vi "LAC Cmd103_Batch Setting_ver2.vi"(6 "R/W (F:Read)":bool, 7 "timeout(ms)":u32=500, 8 "error in":errorcluster, 9 "setting_items":T1={"binary_lvl"=1600, "noise_lvl"=1600, "LM_HiLimit"=1600, "LM_LoLimit"=1600, "LM_Judge"=0, "LM_Judge type"=0, "Circle-radius"=0.0, "Rect-XL"=0.0, "Rect-XH"=0.0, "Rect-YH"=0.0, "Rect-YL"=0.0, "Circle-radius 2"=0.0, "Off-X"=0.0, "Off-Y"=0.0, "Label mode"=64, "Numbering"=64, "Judge label"=64, "Max spot"=3, "Center cal_method"=64, "Average"=64, "Eff Spot mode"=64, "Spot pixel HiLim"=64, "Spot pixel LoLim"=64}, 11 "VISA name in":refnum<visa-resource-name>) -> (0 "error out":errorcluster, 1 "read buffer":string, 3 "VISA name out":refnum<visa-resource-name>)   [LabVIEW 2018]
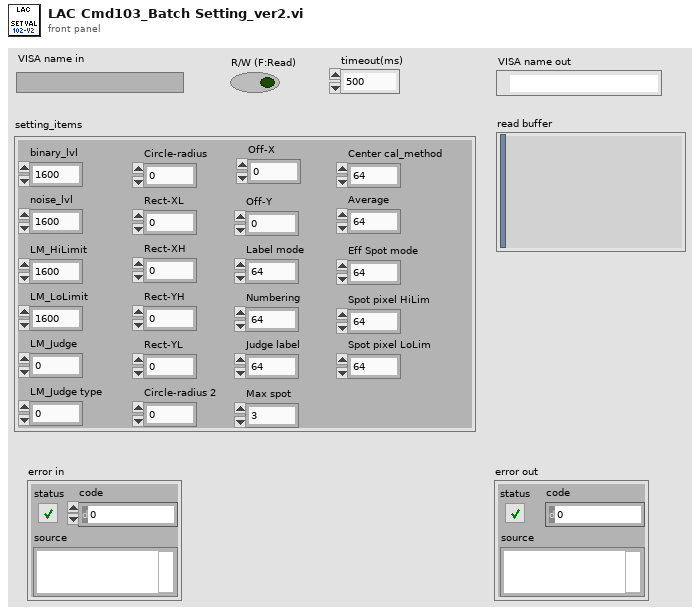
[diagram p1: front panel]
types:
  T1 = cluster{"binary_lvl":u16, "noise_lvl":u16, "LM_HiLimit":u16, "LM_LoLimit":u16, "LM_Judge":u8, "LM_Judge type":u8, "Circle-radius":dbl, "Rect-XL":dbl, "Rect-XH":dbl, "Rect-YH":dbl, "Rect-YL":dbl, "Circle-radius 2":dbl, "Off-X":dbl, "Off-Y":dbl, "Label mode":u8, "Numbering":u8, "Judge label":u8, "Max spot":u8, "Center cal_method":u8, "Average":u8, "Eff Spot mode":u8, "Spot pixel HiLim":u16, "Spot pixel LoLim":u16}
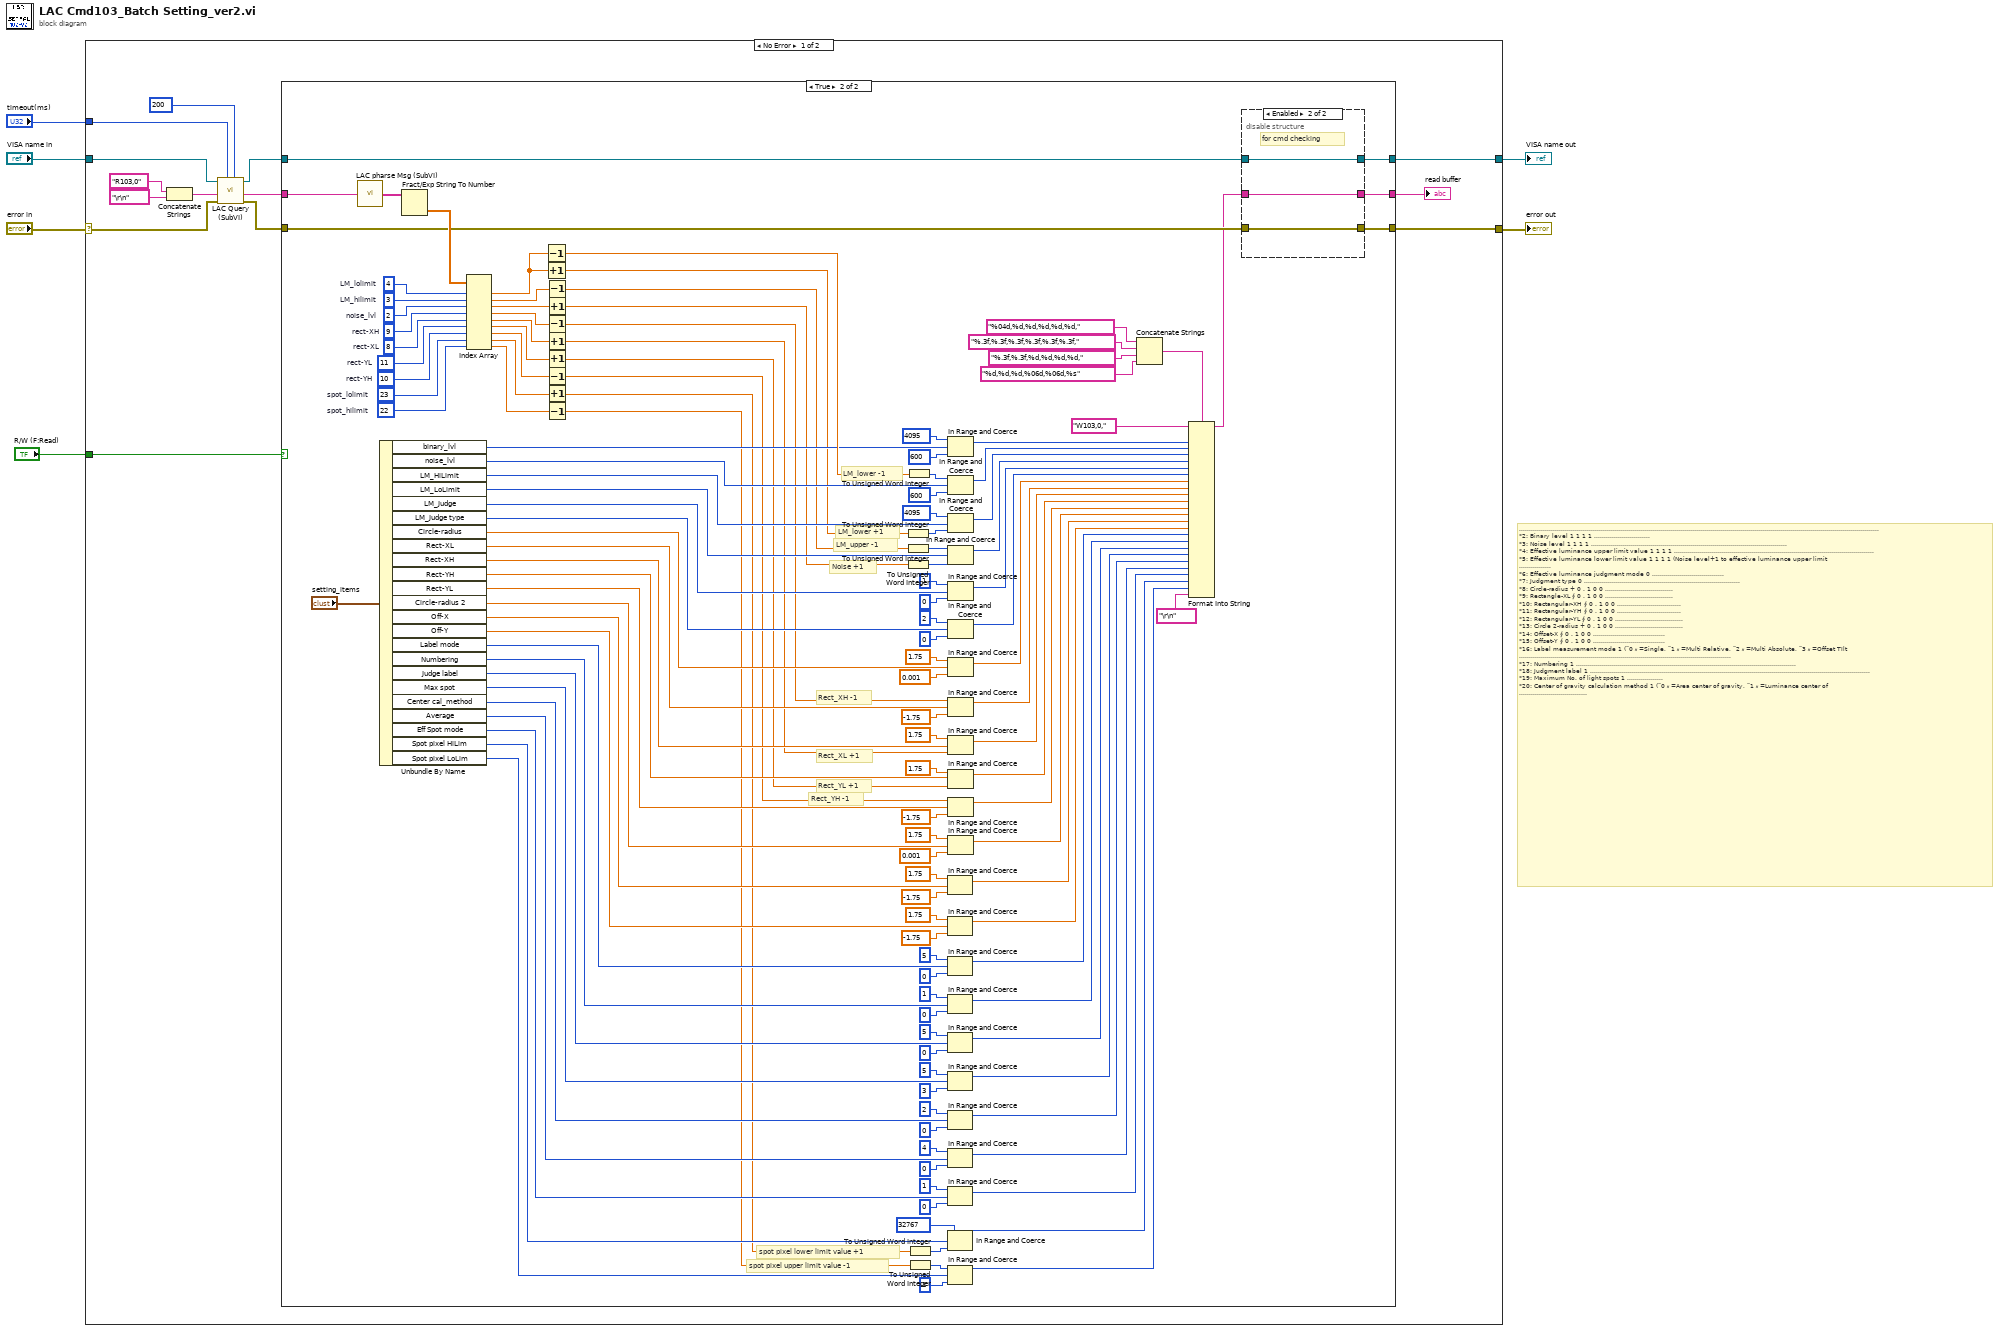
[diagram p0: block diagram]
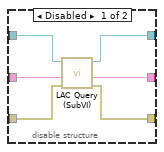
[diagram p3: hidden frame]
diagram:
  # "....................................................................................................................................................................................\n*2: Binary level 1 1 1 1 ............................\n*3: Noise level 1 1 1 1 ..................................................................................................\n*4: Effective luminance upper limit value 1 1 1 1 ....................................................................................................\n*5: Effective luminance lower limit value 1 1 1 1 (Noise level+1 to effective luminance upper limit\n................\n*6: Effective luminance judgment mode 0 ....................................\n*7: Judgment type 0 ..............................................................................\n*8: Circle-radius + 0 . 1 0 0 ..................................\n*9: Rectangle-XL ∮ 0 . 1 0 0 ..................................\n*10: Rectangular-XH ∮ 0 . 1 0 0 ................................\n*11: Rectangular-YH ∮ 0 . 1 0 0 ................................\n*12: Rectangular-YL ∮ 0 . 1 0 0 ..................................\n*13: Circle 2-radius + 0 . 1 0 0 ..................................\n*14: Offset-X ∮ 0 . 1 0 0 ....................................\n*15: Offset-Y ∮ 0 . 1 0 0 ....................................\n*16: Label measurement mode 1 (¨0〃=Single, ¨1〃=Multi Relative, ¨2〃=Multi Absolute, ¨3〃=Offset TIlt\n..........................................................................................................\n*17: Numbering 1 ..............................................................................................................\n*18: Judgment label 1 ............................................................................................................................................\n*19: Maximum No. of light spots 1 ..................\n*20: Center of gravity calculation method 1 (¨0〃=Area center of gravity, ¨1〃=Luminance center of\n........................................................\n*21: Average 1 ..............................................................................................................................\n*22: Effective light spot size mode 1 ....................................\n*23: Effective light spot pixel upper limit value 1 1 1 1 1 1 (Effective light spot pixel lower limit\n..................................\n*24: Effective light spot pixel lower limit value 1 1 1 1 1 1 (1 to Effective light spot pixel upper limit\n................"
  n1 = case shown="No Error" "error in" {
    selector: "error in" -> [w19 w167]
    tunnel: [w9 w166] -> w6
    tunnel: [w8 w167] -> w5
    tunnel: "timeout(ms)" -> [w20 _]
    tunnel: "R/W (F:Read)" -> [w14 _]
    tunnel: "VISA name in" -> [w10 w166]
    frame No Error {
      n2 = Concatenate Strings("R103,0" ("string"), "\r\n" ("write buffer")) -> (w16:string)
      n3 = call "LAC Query (SubVI).vi"("interval(ms)"=200, "timeout(ms)"=w20, "error in"=w19, "Command"=w16, "VISA name in"=w10) -> ("error out"=w12:errorcluster, "read buffer"=w11:string, "VISA name out"=w13:refnum<visa-resource-name>)  [unwired: 4 in]
      n4 = case shown="True" w14 {
        tunnel: w13 -> [w22 w33]
        tunnel: w12 -> [w23 w36]
        tunnel: w11 -> [w21 w35]
        tunnel: [w23 w32] -> w8
        tunnel: [w22 w31] -> w9
        tunnel: [w21 w29] -> w7
        frame False {
        }
        frame True {
          w45 = 22  # spot_hilimit
          w46 = 23  # spot_lolimit
          w52 = 10  # rect-YH
          w53 = 11  # rect-YL
          w54 = 8  # rect-XL
          w55 = 9  # rect-XH
          w28 = 4  # LM_lolimit
          w155 = 3  # LM_hilimit
          w27 = 2  # noise_lvl
          # "LM_lower -1"
          # "LM_lower +1"
          # "LM_upper -1"
          # "Noise +1"
          # "Rect_XH -1"
          # "Rect_XL +1"
          # "Rect_YL +1"
          # "Rect_YH -1"
          # "spot pixel upper limit value -1"
          # "spot pixel lower limit value +1"
          n5 = call "LAC pharse Msg (SubVI).vi"("result"=w35) -> ("array out"=w34:string[])
          n6 = Unbundle By Name("setting_items") -> ("binary_lvl"=w85:u16, "noise_lvl"=w84:u16, "LM_HiLimit"=w83:u16, "LM_LoLimit"=w82:u16, "LM_Judge"=w81:u8, "LM_Judge type"=w80:u8, "Circle-radius"=w79:dbl, "Rect-XL"=w78:dbl, "Rect-XH"=w77:dbl, "Rect-YH"=w76:dbl, "Rect-YL"=w75:dbl, "Circle-radius 2"=w74:dbl, "Off-X"=w73:dbl, "Off-Y"=w72:dbl, "Label mode"=w71:u8, "Numbering"=w70:u8, "Judge label"=w69:u8, "Max spot"=w68:u8, "Center cal_method"=w67:u8, "Average"=w66:u8, "Eff Spot mode"=w65:u8, "Spot pixel HiLim"=w64:u16, "Spot pixel LoLim"=w63:u16)
          n7 = Fract/Exp String To Number(string=w34) -> (number=w156:dbl[])  [unwired: 3 in, 1 out]
          n8 = Index Array(array=w156, index #1=w28, index #2=w155, index #3=w27, index #4=w55, index #5=w54, index #6=w53, index #7=w52, index #8=w46, index #9=w45) -> (element #1=w26:dbl, element #2=w154:dbl, element #3=w25:dbl, element #4=w56:dbl, element #5=w51:dbl, element #6=w50:dbl, element #7=w49:dbl, element #8=w48:dbl, element #9=w47:dbl)
          n9 = Decrement(x=w26) -> (x-1=w88:dbl)
          n10 = Increment(x=w26) -> (x+1=w61:dbl)
          n11 = Decrement(x=w154) -> (x-1=w57:dbl)
          n12 = Increment(x=w25) -> (x+1=w58:dbl)
          n13 = Decrement(x=w56) -> (x-1=w38:dbl)
          n14 = Increment(x=w51) -> (x+1=w39:dbl)
          n15 = Increment(x=w50) -> (x+1=w40:dbl)
          n16 = Decrement(x=w49) -> (x-1=w24:dbl)
          n17 = Increment(x=w48) -> (x+1=w43:dbl)
          n18 = Decrement(x=w47) -> (x-1=w44:dbl)
          n19 = To Unsigned Word Integer(number=w61) -> (unsigned 16bit integer=w62:u16)
          n20 = To Unsigned Word Integer(number=w57) -> (unsigned 16bit integer=w60:u16)
          n21 = To Unsigned Word Integer(number=w58) -> (unsigned 16bit integer=w59:u16)
          n22 = To Unsigned Word Integer(number=w88) -> (unsigned 16bit integer=w87:u16)
          n23 = To Unsigned Word Integer(number=w43) -> (unsigned 16bit integer=w41:u16)
          n24 = To Unsigned Word Integer(number=w44) -> (unsigned 16bit integer=w42:u16)
          n25 = In Range and Coerce(upper limit=1.75 ("y"), x=w73, lower limit=-1.75) -> (coerced(x)=w143:dbl)  [unwired: 1 out]
          n26 = In Range and Coerce(upper limit=1.75 ("y"), x=w72, lower limit=-1.75) -> (coerced(x)=w144:dbl)  [unwired: 1 out]
          n27 = In Range and Coerce(upper limit=u8 5 ("y"), x=w71, lower limit=u8 0) -> (coerced(x)=w145:u8)  [unwired: 1 out]
          n28 = In Range and Coerce(upper limit=u8 1 ("y"), x=w70, lower limit=u8 0) -> (coerced(x)=w146:u8)  [unwired: 1 out]
          n29 = In Range and Coerce(upper limit=u8 5 ("y"), x=w69, lower limit=u8 0) -> (coerced(x)=w147:u8)  [unwired: 1 out]
          n30 = In Range and Coerce(upper limit=u8 5 ("y"), x=w68, lower limit=u8 3) -> (coerced(x)=w148:u8)  [unwired: 1 out]
          n31 = In Range and Coerce(upper limit=u8 2 ("y"), x=w67, lower limit=u8 0) -> (coerced(x)=w149:u8)  [unwired: 1 out]
          n32 = In Range and Coerce(upper limit=u8 4 ("y"), x=w66, lower limit=u8 0) -> (coerced(x)=w150:u8)  [unwired: 1 out]
          n33 = In Range and Coerce(upper limit=u8 1 ("y"), x=w65, lower limit=u8 0) -> (coerced(x)=w151:u8)  [unwired: 1 out]
          n34 = In Range and Coerce(upper limit=u16 32767 ("y"), x=w64, lower limit=w41) -> (coerced(x)=w152:u16)  [unwired: 1 out]
          n35 = In Range and Coerce(upper limit=w42, x=w63, lower limit=u16 1 ("y")) -> (coerced(x)=w153:u16)  [unwired: 1 out]
          n36 = In Range and Coerce(upper limit=u16 4095 ("y"), x=w85, lower limit=u16 600) -> (coerced(x)=w131:u16)  [unwired: 1 out]
          n37 = In Range and Coerce(upper limit=w87, x=w84, lower limit=u16 600) -> (coerced(x)=w132:u16)  [unwired: 1 out]
          n38 = In Range and Coerce(upper limit=u16 4095 ("y"), x=w83, lower limit=w62) -> (coerced(x)=w133:u16)  [unwired: 1 out]
          n39 = In Range and Coerce(upper limit=w60, x=w82, lower limit=w59) -> (coerced(x)=w134:u16)  [unwired: 1 out]
          n40 = In Range and Coerce(upper limit=u8 1 ("y"), x=w81, lower limit=u8 0) -> (coerced(x)=w135:u8)  [unwired: 1 out]
          n41 = In Range and Coerce(upper limit=u8 2 ("y"), x=w80, lower limit=u8 0) -> (coerced(x)=w136:u8)  [unwired: 1 out]
          n42 = In Range and Coerce(upper limit=1.75 ("y"), x=w79, lower limit=0.001) -> (coerced(x)=w137:dbl)  [unwired: 1 out]
          n43 = In Range and Coerce(upper limit=w38, x=w78, lower limit=-1.75) -> (coerced(x)=w138:dbl)  [unwired: 1 out]
          n44 = In Range and Coerce(upper limit=1.75 ("y"), x=w77, lower limit=w39) -> (coerced(x)=w139:dbl)  [unwired: 1 out]
          n45 = In Range and Coerce(upper limit=1.75 ("y"), x=w76, lower limit=w40) -> (coerced(x)=w140:dbl)  [unwired: 1 out]
          n46 = In Range and Coerce(upper limit=w24, x=w75, lower limit=-1.75) -> (coerced(x)=w141:dbl)  [unwired: 1 out]
          n47 = In Range and Coerce(upper limit=1.75 ("y"), x=w74, lower limit=0.001) -> (coerced(x)=w142:dbl)  [unwired: 1 out]
          n48 = Concatenate Strings("%04d,%d,%d,%d,%d,%d," ("format string"), "%.3f,%.3f,%.3f,%.3f,%.3f,%.3f," ("string"), "%.3f,%.3f,%d,%d,%d,%d," ("string"), "%d,%d,%d,%06d,%06d,%s" ("format string")) -> (w130:string)
          n49 = Format Into String(format string=w130, initial string="W103,0," ("string"), w131, w132, w133, w134, w135, w136, w137, w138, w139, w140, w141, w142, w143, w144, w145, w146, w147, w148, w149, w150, w151, w152, w153, "\r\n" ("write buffer")) -> (resulting string=w30:string)  [unwired: 1 in, 1 out]
          n50 = disable-structure shown="Enabled" {
            disable-tunnel: w36 -> [w162 w163]
            disable-tunnel: w33 -> [w161 w165]
            disable-tunnel: [w160 w163] -> w32
            disable-tunnel: [w159 w165] -> w31
            disable-tunnel: w30 -> [w158 w164]
            disable-tunnel: [w157 w164] -> w29
            frame Disabled {
              n51 = call "LAC Query (SubVI).vi"("error in"=w162, "Command"=w158, "VISA name in"=w161) -> ("error out"=w160:errorcluster, "read buffer"=w157:string, "VISA name out"=w159:refnum<visa-resource-name>)  [unwired: 6 in]
            }
            frame Enabled {
              # "for cmd checking"
            }
          }
        }
      }
      "read buffer" <- w7
    }
    frame Error {
    }
  }
  "VISA name out" <- w6
  "error out" <- w5
